vi "readReg.vi"(7 "I2C Channel":u8, 8 "error in":errorcluster, 9 "Bytes To Read":u8, 10 "I2C Slave Address":u8, 11 "LINX Resource in":T1) -> (0 "error out":errorcluster, 2 "Bytes Read":u8[](array[numeric]), 3 "LINX Resource out":T1)   [LabVIEW 2017]
uses:
  <vilib>/myRIO/Instrument Drivers/Onboard IO/I2C/I2C.lvlib
  <vilib>/myRIO/Instrument Drivers/Onboard IO/I2C/typedefs/I2C Transfer Rate.ctl
  <vilib>/myRIO/Instrument Drivers/Onboard IO/I2C/typedefs/I2C User Configuration.ctl
  <vilib>/myRIO/Express VI/Onboard IO/I2C/I2C Express VI.xnode
  <vilib>/myRIO/Instrument Drivers/Onboard IO/I2C/typedefs/I2C Configuration.ctl
  <vilib>/myRIO/Common/Instrument Driver Framework/myRIO v1.0/I2C/typedefs/I2C Channels Enum.ctl
  <vilib>/myRIO/Common/Instrument Driver Framework/Utilities/typedefs/Generic FPGA Reference.ctl
  <vilib>/myRIO/Common/Instrument Driver Framework/Utilities/typedefs/myRIO v1.0 Reference.ctl
  <vilib>/myRIO/Common/Instrument Driver Framework/Utilities/typedefs/Hardware Version Enum.ctl
  <vilib>/myRIO/Common/Instrument Driver Framework/Utilities/typedefs/myRIO Generic Hardware Reference.ctl
  <vilib>/myRIO/Instrument Drivers/Onboard IO/I2C/typedefs/I2C Reference.ctl
  <vilib>/myRIO/Instrument Drivers/Onboard IO/I2C/vis/myRIO I2C Open.xnode
  <vilib>/myRIO/Common/Instrument Driver Framework/Utilities/vis/Is FPGA Ref Available.vi
  <vilib>/myRIO/Common/Instrument Driver Framework/myRIO v1.0/I2C/vis/myRIO v1.1 Open I2C.vi
  <vilib>/userdefined/High Color/nirio_resource_hc.ctl
  <vilib>/MakerHub/LINX/Private/Type Defs/Platform.ctl
  <vilib>/MakerHub/LINX/Private/Type Defs/Interface.ctl
  <vilib>/MakerHub/LINX/Private/Device/Type Defs/TCP Config.ctl
  <vilib>/MakerHub/LINX/Private/Device/Type Defs/Channels.ctl
  <vilib>/MakerHub/LINX/Private/Device/Type Defs/LINX Device Config.ctl
  <vilib>/MakerHub/LINX/Private/Type Defs/LINX Ref.ctl
panel:
  in  "I2C Impl.":enum16{"LINX", "myRIO Express", "myRIO subVIs"}(ring)
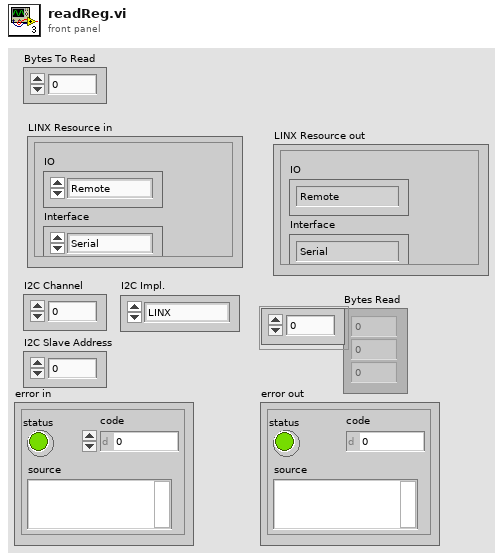
[diagram p1: front panel]
types:
  T1 = typedef "LMH-LINX.lvlib/LINX Ref.ctl" = cluster{"IO":T2, "Interface":T3, "LINX Device Config":T4}
  T2 = typedef "LMH-LINX.lvlib/Platform.ctl" = enum16{"Remote", "Local"}
  T3 = typedef "LMH-LINX.lvlib/Interface.ctl" = enum16{"Serial", "TCP"}
  T4 = typedef "LMH-LINX.lvlib/Device.lvlib/LINX Device Config.ctl" = cluster{"Interface":T3, "COM Port":refnum<visa-resource-name>, "TCP Configuration":T5, "Device Family":u8, "Device ID":u8, "Device Name":string, "TCP Ref":refnum<k5>, "Channels":T6}
  T5 = typedef "LMH-LINX.lvlib/Device.lvlib/TCP Config.ctl" = cluster{"IP Address":string, "Port":u16}
  T6 = typedef "LMH-LINX.lvlib/Channels.ctl" = cluster{"DI":u8[], "DO":u8[], "AI":u8[], "AO":u8[], "PWM":u8[], "QE":u8[], "UART":u8[], "I2C 2":u8[], "SPI":u8[], "CAN":u8[], "Servo":u8[], "AI Ref (V)":dbl, "AI Resolution (Bits)":u8, "AO Ref (V)":dbl, "AO Resolution (Bits)":u8}
  T7 = typedef "I2C.lvlib/I2C Reference.ctl" = cluster{"myRIO Reference":T8, "I2C Channels Enum":T12, "I2C Configuration":T13}
  T8 = typedef "myRIO Generic Hardware Reference.ctl" = cluster{"myRIO Model":T9, "myRIO Hardware Reference":T10}
  T9 = typedef "Hardware Version Enum.ctl" = enum16{"Unknown", "myRIO-1900", "myRIO-1950", "roboRIO", "NI ELVIS RIO CM", "ELVIS III"}
  T10 = typedef "myRIO v1.0 Reference.ctl" = cluster{"Generic FPGA Reference":T11, "Allow multiple opens":bool}
  T11 = typedef "Generic FPGA Reference.ctl" = refnum<k20>
  T12 = typedef "I2C Channels Enum.ctl" = enum16{"Not Connected", "A/I2C", "B/I2C", "I2C/I2C"}
  T13 = typedef "I2C.lvlib/I2C Configuration.ctl" = cluster{"I2C Transfer Rate":T14}
  T14 = typedef "I2C.lvlib/I2C Transfer Rate.ctl" = enum16{"Standard mode (100 kbps)", "Fast mode (400 kbps)"}
  T15 = typedef "I2C.lvlib/I2C User Configuration.ctl" = cluster{"I2C Transfer Rate":T14}
  T16 = typedef "nirio_resource_hc.ctl" = tag
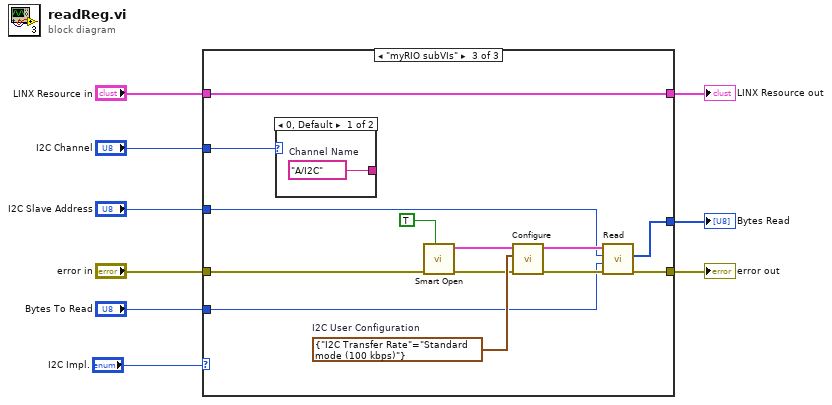
[diagram p0: block diagram]
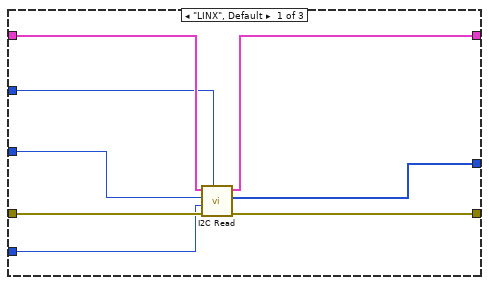
[diagram p2: hidden frame]
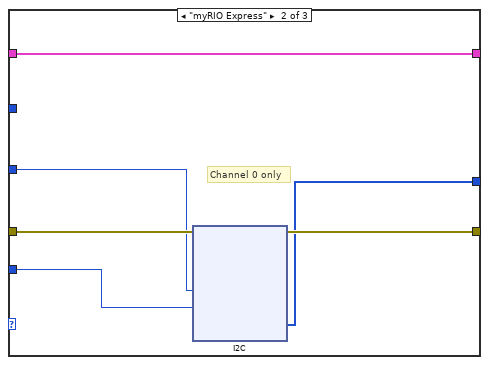
[diagram p3: hidden frame]
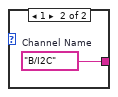
[diagram p4: hidden frame]
diagram:
  n1 = case shown="\"myRIO subVIs\"" "I2C Impl." {
    tunnel: [w15 w20 w74] -> w9
    tunnel: "error in" -> [w17 w22 w69]
    tunnel: [w16 w21 w68] -> w7
    tunnel: "I2C Slave Address" -> [w12 w19 w67]
    tunnel: "Bytes To Read" -> [w10 w18 w66]
    tunnel: "I2C Channel" -> [w11 _ w65]
    tunnel: "LINX Resource in" -> [w13 w23 w64]
    tunnel: [w14 w23 w64] -> w1
    frame "LINX", Default {
      n2 = call <vilib>:"I2C Read.vi"("I2C Channel"=w11, "Error In"=w17, "Bytes To Read"=w10, "I2C Slave Address (0)"=w12, "LINX Resource"=w13) -> ("Error Out"=w16:errorcluster, "Data"=w15:u8[], "LINX Resource"=w14:T1)  [unwired: 4 in]
    }
    frame "myRIO Express" {
      # "Channel 0 only"
      n3 = xnode "I2C"("Slave Address (7-bit)"=w19, "Byte Count"=w18, "error in (no error)"=w22) -> ("Bytes Read"=w20:u8[], "error out"=w21:errorcluster)
    }
    frame "myRIO subVIs" {
      w75 = T15 {"I2C Transfer Rate"=enum."Standard mode (100 kbps)"}  # I2C User Configuration
      n4 = case shown="0, Default" w65 {
        tunnel: [w76 w77] -> _
        frame 0, Default {
          w76 = tag "A/I2C"  # Channel Name
        }
        frame 1 {
          w77 = tag "B/I2C"  # Channel Name
        }
      }
      n5 = call <vilib>:"Smart Open.vi"("Allow multiple opens?"=TRUE, "error in (no error)"=w69) -> ("error out"=w72:errorcluster, "I2C Ref Out"=w73:T7)  [unwired: 8 in]
      n6 = call <vilib>:"Configure.vi"("error in (no error)"=w72, "I2C User Configuration"=w75, "I2C Ref In"=w73) -> ("error out"=w70:errorcluster, "I2C Ref Out"=w71:T7)  [unwired: 7 in]
      n7 = call <vilib>:"Read.vi"("error in (no error)"=w70, "Byte Count"=w66, "Slave Address (7-bit)"=w67, "I2C Ref In"=w71) -> ("error out"=w68:errorcluster, "Bytes Read"=w74:u8[])  [unwired: 4 in, 1 out]
    }
  }
  "error out" <- w7
  "LINX Resource out" <- w1
  "Bytes Read" <- w9
